vi "Destroy Data Channels.vi"(8 "error in":errorcluster, 11 "Node in":refnum<class "BLS Power Supply Template.lvclass">) -> (0 "error out":errorcluster, 3 "Node out":refnum<class "BLS Power Supply Template.lvclass">)   [LabVIEW 2023, in "BLS Power Supply Template.lvlib" / "BLS Power Supply Template.lvclass"]
uses:
  BLS Power Supply Template.lvclass
  BLS Power Supply Template.lvclass/BLS Power Supply Template.ctl
  <vilib>/ADAS Replay HIL/AdasHilServices/AdasHilServices Fill In Error Info Ex.vi
  <vilib>/ADAS Replay HIL/AdasHilServices/AdasHilChannelServices.lvlib
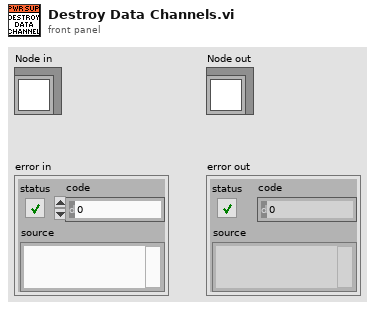
[diagram p1: front panel]
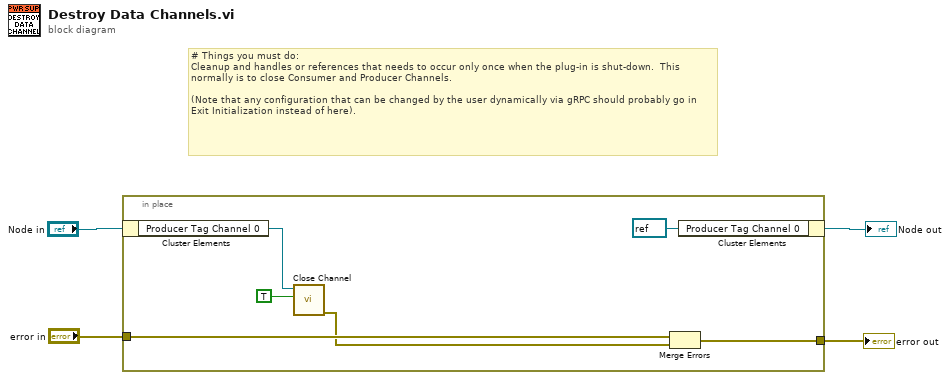
[diagram p0: block diagram]
diagram:
  # "# Things you must do:\nCleanup and handles or references that needs to occur only once when the plug-in is shut-down.  This normally is to close Consumer and Producer Channels.   \n\n(Note that any configuration that can be changed by the user dynamically via gRPC should probably go in Exit Initialization instead of here)."
  n1 = in-place {
    in-place-border: [w7] -> w1
    in-place-border: "error in" -> [w9]
    n2 = in-place-cluster #1("Node in") -> ("Producer Tag Channel 0"=w10:refnum<k21>)
    n3 = call <vilib>:"Close Channel.vi"("Force Destroy? (F)"=TRUE ("force destroy? (F)"), "ADAS HIL Channel"=w10) -> ("error out"=w8:errorcluster)  [unwired: 9 in]
    n4 = Merge Errors(w9, w8) -> (w7:errorcluster)
    n5 = in-place-cluster #1("Producer Tag Channel 0"=refnum<k21> refnum ("Producer Tag Channel")) -> (→"Node out":refnum<class "BLS Power Supply Template.lvclass">)
  }
  "error out" <- w1
